vi "Write iName.vi"(8 "error in (no error)":errorcluster, 10 "iName":string, 11 "Ancestral Actor in":refnum<class "Ancestral Actor.lvclass">) -> (0 "error out":errorcluster, 3 "Ancestral Actor out":refnum<class "Ancestral Actor.lvclass">)   [LabVIEW 2016, in "Stream Actor.lvlib" / "Ancestral Actor.lvclass"]
doc: "--\nCopyright © 2017 Composed SystemsI All rights reserved.\n\nAuthor: Jon McBee <jon.mcbee@composed.io>\n\nThis library is provided \"AS IS\" ,WITHOUT WARRANTIES OR\nCONDITIONS OF ANY KIND, either express or implied.\n\nComposed Systems -- composed.io\n\nStream 0.0.1.1\nJon McBee - Composed Systems\nCopyright (c) 2017, Composed Systems"
uses:
  <userlib>/Composed Systems/Stream/Actor/Actor Class/Ancestral Actor.lvclass
  <userlib>/Composed Systems/Stream/Actor/Actor Class/Ancestral Actor.lvclass/Ancestral Actor.ctl
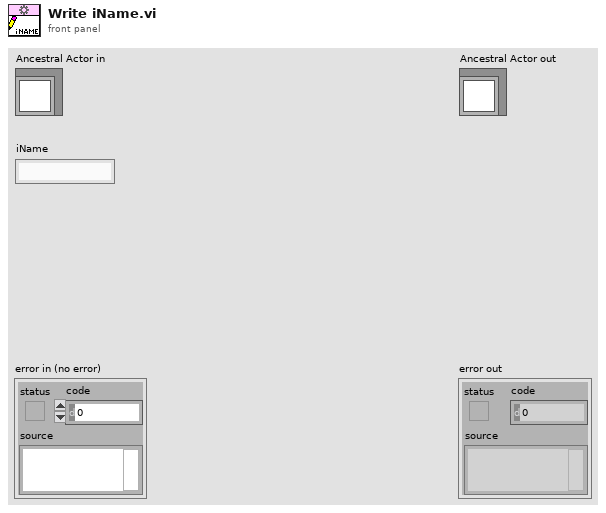
[diagram p1: front panel]
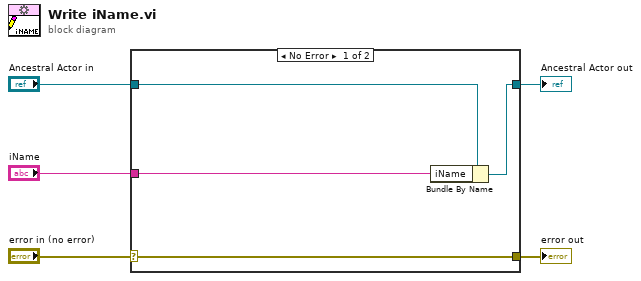
[diagram p0: block diagram]
diagram:
  n1 = case shown="No Error" "error in (no error)" {
    selector: "error in (no error)" -> [w9 w10]
    tunnel: [w9 w10] -> w4
    tunnel: [w7 w11] -> w2
    tunnel: "Ancestral Actor in" -> [w8 w11]
    tunnel: "iName" -> [w6 _]
    frame No Error {
      n2 = Bundle By Name(cluster=w8, "iName"=w6) -> (w7:refnum<class "Ancestral Actor.lvclass">)
    }
    frame Error {
    }
  }
  "error out" <- w4
  "Ancestral Actor out" <- w2
